vi "Save_2D_Array_Dialog.vi"(0 "2D data":dbl[][](array[numeric]) format="%0.2f") -> ()   [LabVIEW 2019]
doc: "Sub-VI for saving a 2D array to some directory, storing the data in the file Filename\n\nData is saved with 10 decimal places by default. \n\nR. Sheehan 6 - 1 - 2017"
uses:
  <vilib>/Utility/file.llb/Write Delimited Spreadsheet (DBL).vi
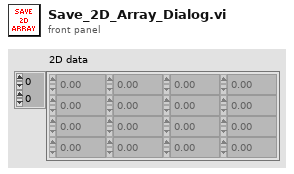
[diagram p1: front panel]
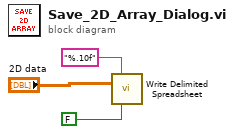
[diagram p0: block diagram]
diagram:
  n1 = call-poly <vilib>:"Write Delimited Spreadsheet.vi"("format (%.3f)"="%.10f", "2D data"="2D data", "transpose? (no:F)"=FALSE) -> ()  [unwired: 11 in, 2 out]
